vi "shutdown_request Message_Init.vi"(8 "error in (no error)":errorcluster, 11 "Object in":refnum<class "shutdown_request Message.lvclass">) -> (0 "error out":errorcluster, 3 "object out":refnum<class "shutdown_request Message.lvclass">)   [LabVIEW 2018, in "ClientMessaging.lvlib" / "shutdown_request Message.lvclass"]
uses:
  shutdown_request Message.lvclass
  C:/Users/gavin/Documents/Programming/LabVIEW/JuPyterClient/Base Classes/Request Message/Request Message.lvclass
  shutdown_request Message.lvclass/shutdown_request Message.ctl
  Base Classes/Request Message/Request Message.lvclass
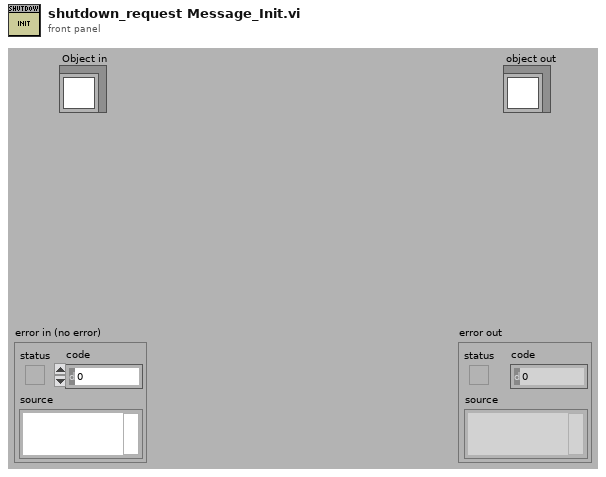
[diagram p1: front panel]
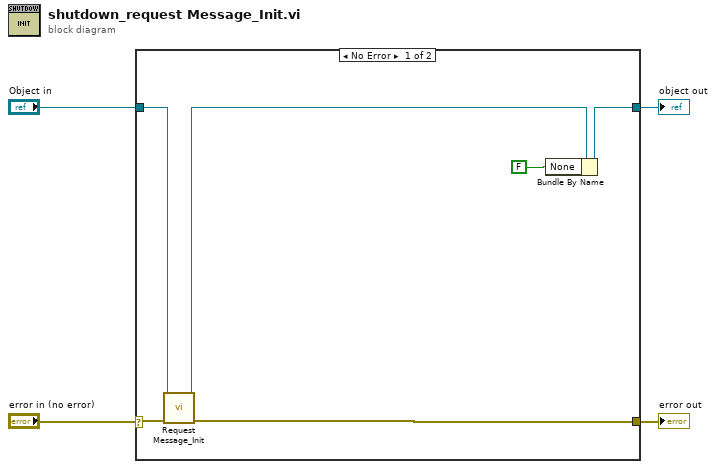
[diagram p0: block diagram]
diagram:
  n1 = case shown="No Error" "error in (no error)" {
    selector: "error in (no error)" -> [w8 w11]
    tunnel: [w10 w12] -> w4
    tunnel: "Object in" -> [w6 w12]
    tunnel: [w7 w11] -> w1
    frame No Error {
      n2 = call "Request Message_Init.vi"("error in (no error)"=w8, "object in"=w6) -> ("error out"=w7:errorcluster, "object out"=w5:refnum<class "shutdown_request Message.lvclass">)  [unwired: 8 in]
      n3 = Bundle By Name(cluster=w5, "None"=FALSE) -> (w10:refnum<class "shutdown_request Message.lvclass">)
    }
    frame Error {
    }
  }
  "object out" <- w4
  "error out" <- w1
